vi "HEWH Scan Rate Loop Trigger.vi"(10 "Scan Rate (Seconds)":i16=3, 11 "Array Index Input":i16) -> (1 "output array":bool[](array[boolean]), 2 "Loop Trigger":bool, 3 "Array Index Output":i16)   [LabVIEW 2020]
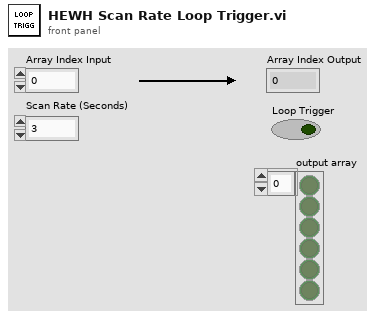
[diagram p1: front panel]
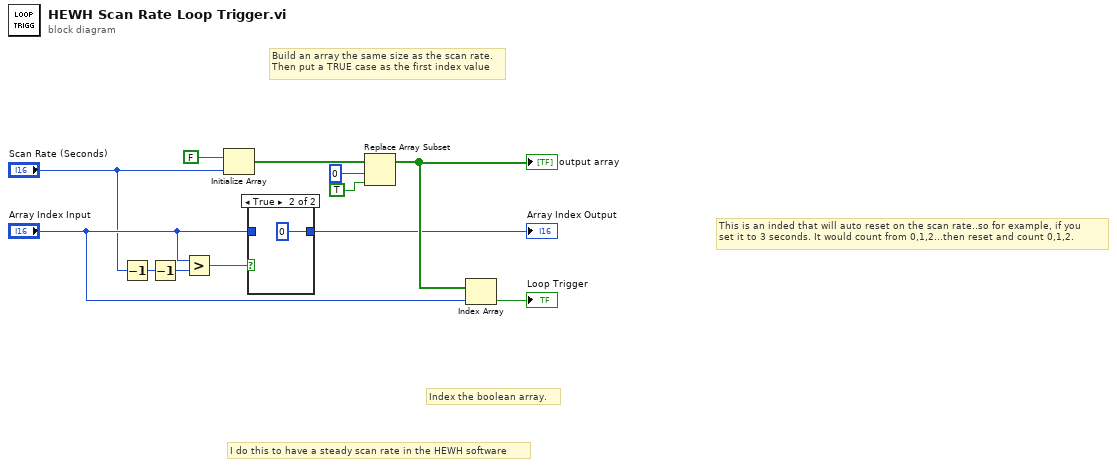
[diagram p0: block diagram]
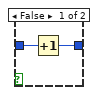
[diagram p2: hidden frame]
diagram:
  # "I do this to have a steady scan rate in the HEWH software"
  # "Index the boolean array."
  # "Build an array the same size as the scan rate.\nThen put a TRUE case as the first index value"
  # "This is an inded that will auto reset on the scan rate..so for example, if you\nset it to 3 seconds. It would count from 0,1,2...then reset and count 0,1,2."
  n1 = Decrement(x="Scan Rate (Seconds)") -> (x-1=w8:i16)
  n2 = Decrement(x=w8) -> (x-1=w9:i16)
  n3 = Greater?(x="Array Index Input", y=w9) -> (0:w3:bool)
  n4 = Initialize Array(FALSE, "Scan Rate (Seconds)") -> (w5:bool[])
  n5 = case shown="True" w3 {
    tunnel: "Array Index Input" -> [w14 _]
    tunnel: [w13 i16 0] -> w2
    frame False {
      n6 = Increment(x=w14) -> (x+1=w13:i16)
    }
    frame True {
    }
  }
  "Array Index Output" <- w2
  n7 = Replace Array Subset(array=w5, new element=TRUE ("new element/subarray"), index=0) -> (w10:bool[])
  "output array" <- w10
  n8 = Index Array(array=w10, index="Array Index Input") -> (element=→"Loop Trigger":bool)
